vi "Set-Image-width.vi"(8 "error in (no error)":errorcluster, 10 "Image width in":i32, 11 "PF_MV1-D1312-240 in":refnum<class "PF_MV1-D1312-240.lvclass">) -> (0 "error out":errorcluster, 1 "Image width delta":i32, 2 "Image width":i32, 3 "PF_MV1-D1312-240 out":refnum<class "PF_MV1-D1312-240.lvclass">)   [LabVIEW 2013, in "CameraVision.lvlib" / "PF_MV1-D1312-240.lvclass"]
uses:
  PF_MV1-D1312-240.lvclass
  Camera.lvclass/Camera.ctl
  Read IMAQ Session.vi
  <userlib>/Photonfocus Toolkit/_Public/SubVIs/pf_Set_Camera_Property_Int.vi
  <userlib>/Photonfocus Toolkit/Photonfocus_Toolkit.lvlib
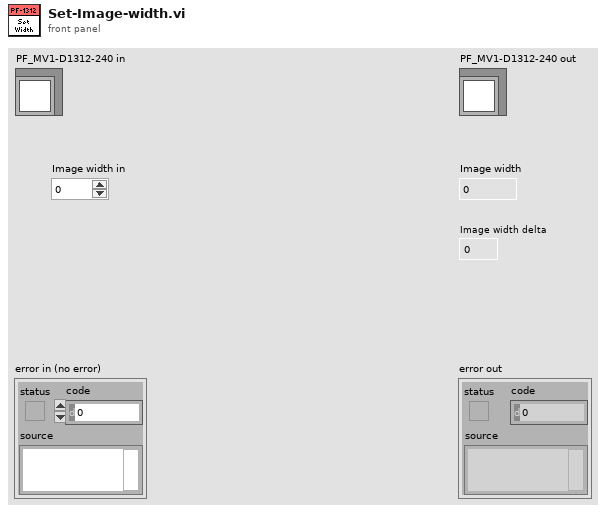
[diagram p1: front panel]
types:
  T1 = cluster{"Max. width":i32, "Max. height":i32, "Step size width":dbl, "Min. width":i32, "Min. height":i32, "Step size height":dbl}
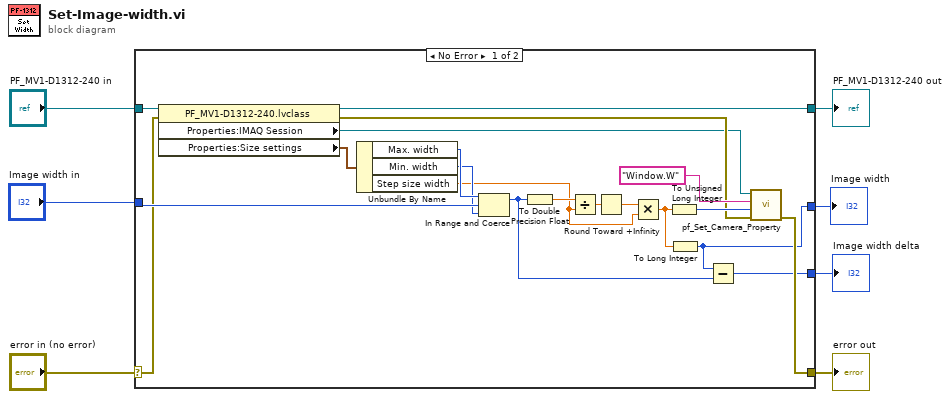
[diagram p0: block diagram]
diagram:
  n1 = case shown="No Error" "error in (no error)" {
    selector: "error in (no error)" -> [w17 w30]
    tunnel: [w27 w30] -> w6
    tunnel: [w16 w29] -> w4
    tunnel: "PF_MV1-D1312-240 in" -> [w18 w29]
    tunnel: "Image width in" -> [w25 w28]
    tunnel: [w21 _] -> w2
    tunnel: [w8 w28] -> w1
    frame No Error {
      n2 = property class="PF_MV1-D1312-240.lvclass"(reference=w18, error in=w17) -> (reference out=w16:refnum<class "PF_MV1-D1312-240.lvclass">, error out=w15:errorcluster, "Properties:IMAQ Session"=w14:refnum<k11>, "Properties:Size settings"=w13:T1)
      n3 = Unbundle By Name(w13) -> ("Max. width"=w12:i32, "Min. width"=w11:i32, "Step size width"=w10:dbl)
      n4 = In Range and Coerce(upper limit=w12, x=w25, lower limit=w11) -> (coerced(x)=w19:i32)  [unwired: 1 out]
      n5 = To Double Precision Float(number=w19) -> (double precision float=w22:dbl)
      n6 = Divide(x=w22, y=w10) -> (x/y=w24:dbl)
      n7 = Round Toward +Infinity(x=w24) -> (ceil(x): smallest int >= x=w23:dbl)
      n8 = Multiply(x=w23, y=w10) -> (x*y=w9:dbl)
      n9 = To Unsigned Long Integer(number=w9) -> (unsigned 32bit integer=w20:u32)
      n10 = To Long Integer(number=w9) -> (32bit integer=w8:i32)
      n11 = Subtract(x=w8, y=w19) -> (x-y=w21:i32)
      n12 = call-poly <userlib>:"pf_Set_Camera_Property.vi"("error in (no error)"=w15, "Property Value"=w20, "Property Name"="Window.W", "IMAQ Session in"=w14) -> ("error out"=w27:errorcluster)  [unwired: 5 in, 2 out]
    }
    frame Error {
    }
  }
  "error out" <- w6
  "PF_MV1-D1312-240 out" <- w4
  "Image width delta" <- w2
  "Image width" <- w1
